vi "Handle Command.vi"(8 "error in (no error)":errorcluster, 9 "params in":variant, 10 "command":string, 11 "Instrument in":refnum<class "Instrument.lvclass">) -> (0 "error out":errorcluster, 1 "processed data":variant, 2 "command out":string, 3 "Instrument out":refnum<class "Instrument.lvclass">)   [LabVIEW 2019, in "Instrument.lvlib" / "Instrument.lvclass"]
doc: "Override to add additional commands supported by your Instrument."
uses:
  Instrument.lvclass
  Typedefs/Instrument.Commands--Enum.ctl
  Typedefs/Instrument.ProtectedCommands--Enum.ctl
  Typedefs/Instrument.SET--cluster.ctl
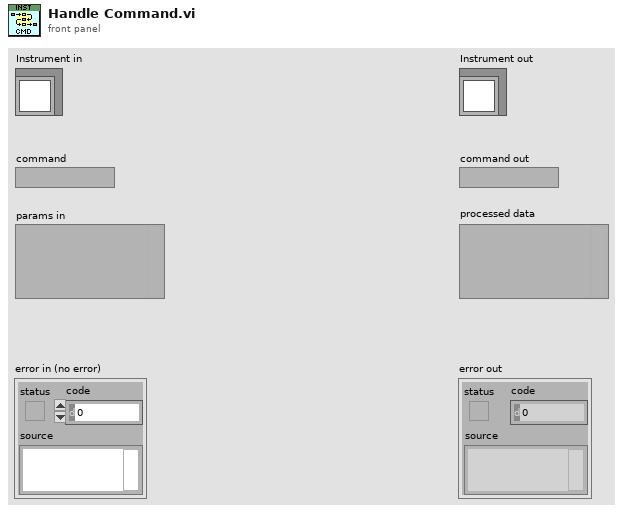
[diagram p1: front panel]
types:
  T1 = typedef "Instrument.lvlib/Instrument.lvclass/Instrument.ProtectedCommands--Enum.ctl" = enum16{"setConfiguration", "setIDN", "setAll", "setAllData"}
  T2 = typedef "Instrument.lvlib/Instrument.lvclass/Instrument.Commands--Enum.ctl" = enum16{"ACK", "HELP", "IDN", "getAll", "getAllData"}
  T3 = typedef "Instrument.lvlib/Instrument.lvclass/Instrument.SET--cluster.ctl" = cluster{"parameter":string, "Data":variant}
  T4 = typedef "Instrument.lvlib/Instrument.lvclass/Instrument.IDN--cluster.ctl" = cluster{"vendor":string, "model":string, "serial":string, "firmware":string}
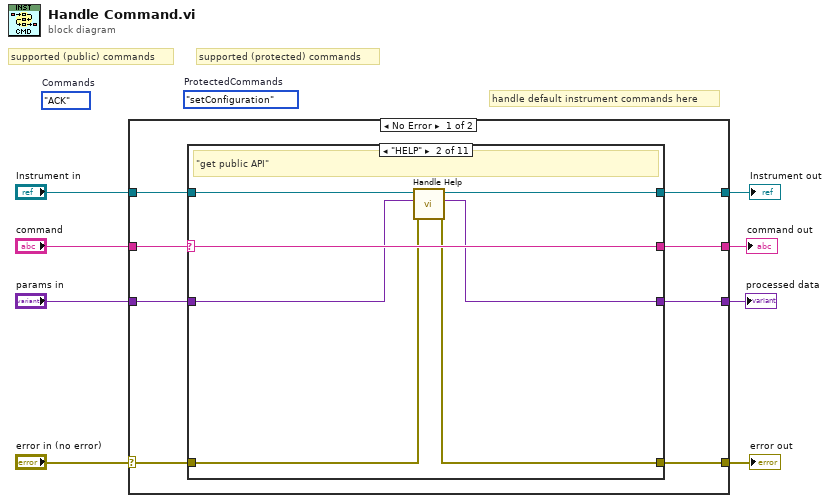
[diagram p0: block diagram]
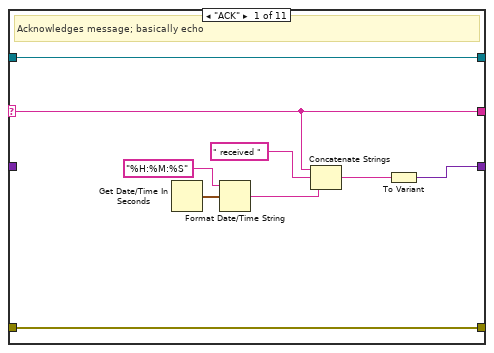
[diagram p2: hidden frame]
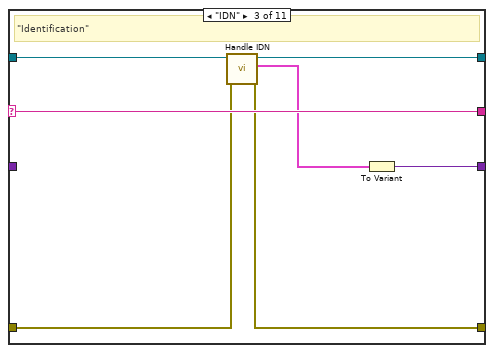
[diagram p3: hidden frame]
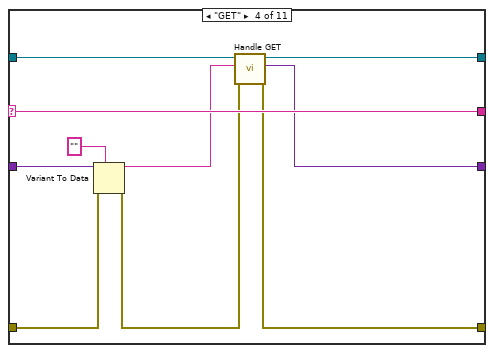
[diagram p4: hidden frame]
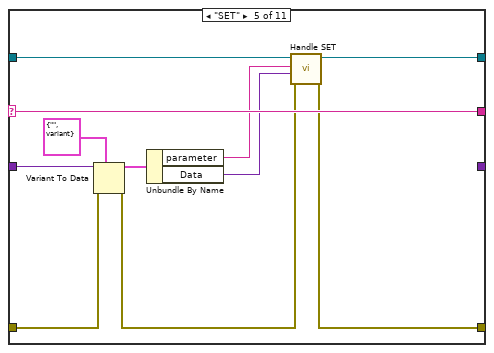
[diagram p5: hidden frame]
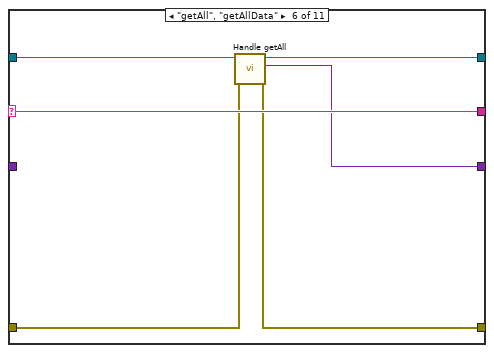
[diagram p6: hidden frame]
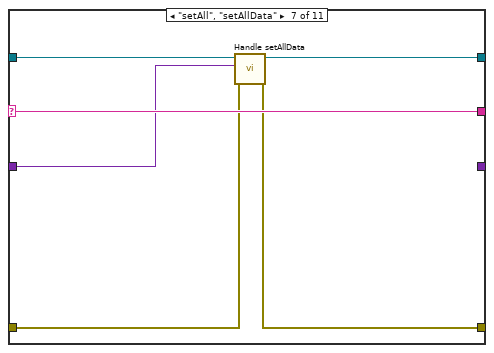
[diagram p7: hidden frame]
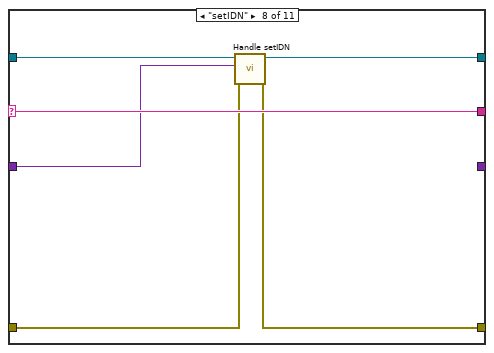
[diagram p8: hidden frame]
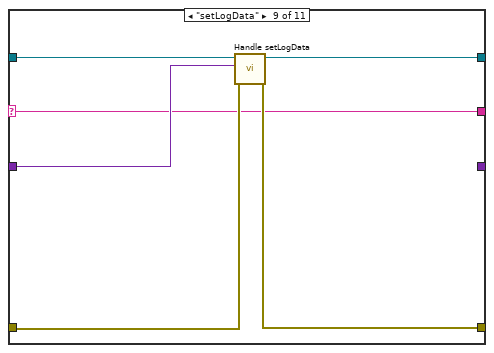
[diagram p9: hidden frame]
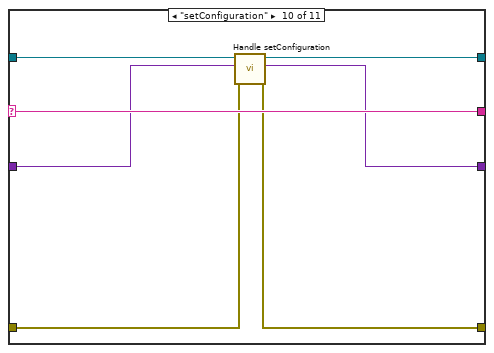
[diagram p10: hidden frame]
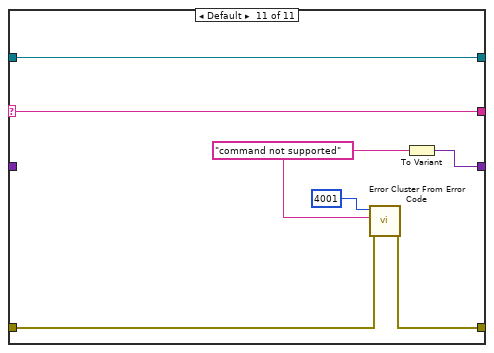
[diagram p11: hidden frame]
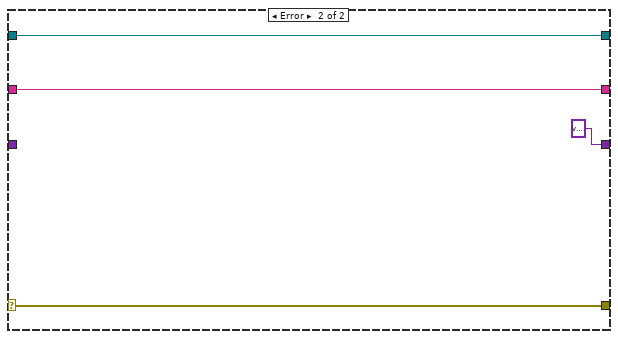
[diagram p12: hidden frame]
diagram:
  (unwired) Instrument.ProtectedCommands--Enum."setConfiguration"  # ProtectedCommands
  (unwired) Instrument.Commands--Enum."ACK"  # Commands
  # "supported (protected) commands"
  # "supported (public) commands"
  # "handle default instrument commands here"
  n1 = case shown="No Error" "error in (no error)" {
    selector: "error in (no error)" -> [w13 w101]
    tunnel: [w12 w101] -> w7
    tunnel: [w15 w100] -> w5
    tunnel: "Instrument in" -> [w16 w100]
    tunnel: "command" -> [w10 w99]
    tunnel: [w14 variant ("error message (\"\")")] -> w4
    tunnel: "params in" -> [w9 _]
    tunnel: [w11 w99] -> w1
    frame No Error {
      n2 = case shown="\"HELP\"" w10 {
        selector: w10 -> [w19 w30 w39 w49 w60 w66 w72 w78 w79 w90 w95]
        tunnel: w16 -> [w25 w32 w36 w47 w58 w63 w71 w76 w84 w87 w97]
        tunnel: [w25 w31 w37 w48 w59 w62 w70 w74 w83 w86 w97] -> w15
        tunnel: [w17 w27 w38 w45 _ w61 _ _ _ w85 w96] -> w14
        tunnel: w13 -> [w22 w29 w33 w41 w53 w65 w69 w77 w81 w89 w93]
        tunnel: [w22 w28 w34 w46 w57 w64 w68 w75 w80 w88 w92] -> w12
        tunnel: [w19 w30 w39 w49 w60 w66 w72 w78 w79 w90 w95] -> w11
        tunnel: w9 -> [_ w26 _ w43 w55 _ w67 w73 w82 w85 _]
        frame "ACK" {
          # "Acknowledges message; basically echo"
          n3 = Get Date/Time In Seconds() -> (seconds since 1Jan1904=w23:timestamp)
          n4 = Format Date/Time String(time format string (%c)="%H:%M:%S", seconds (now)=w23) -> (date/time string=w24:string)  [unwired: 1 in]
          n5 = Concatenate Strings(w19, " received " ("data"), w24) -> (w21:string)
          n6 = To Variant(anything=w21) -> (Variant=w17:variant)
        }
        frame "HELP" {
          # "\"get public API\""
          n7 = call "Handle Help.vi"("error in (no error)"=w29, "Command"=w26, "Instrument in"=w32) -> ("error out"=w28:errorcluster, "Help"=w27:variant, "Instrument out"=w31:refnum<class "Instrument.lvclass">)  [unwired: 6 in]
        }
        frame "IDN" {
          # "\"Identification\""
          n8 = call "Handle IDN.vi"("error in (no error)"=w33, "Instrument in"=w36) -> ("error out"=w34:errorcluster, "IDN"=w35:T4, "Instrument out"=w37:refnum<class "Instrument.lvclass">)  [unwired: 7 in]
          n9 = To Variant(anything=w35) -> (Variant=w38:variant)
        }
        frame "GET" {
          n10 = Variant To Data(error in=w41, type="", Variant=w43) -> (data=w40:string, error out=w42:errorcluster)
          n11 = call-dynamic "Handle GET.vi"("error in (no error)"=w42, "parameter"=w40, "Instrument in"=w47) -> ("error out"=w46:errorcluster, "data out"=w45:variant, "Instrument out"=w48:refnum<class "Instrument.lvclass">)  [unwired: 6 in]
        }
        frame "SET" {
          n12 = Variant To Data(error in=w53, type=T3 {"parameter"="", "Data"=variant} ("GETSET"), Variant=w55) -> (data=w52:T3, error out=w54:errorcluster)
          n13 = Unbundle By Name(w52) -> ("parameter"=w51:string, "Data"=w50:variant)
          n14 = call-dynamic "Handle SET.vi"("error in (no error)"=w54, "data"=w50, "parameter"=w51, "Instrument in"=w58) -> ("error out"=w57:errorcluster, "Instrument out"=w59:refnum<class "Instrument.lvclass">)  [unwired: 5 in, 1 out]
        }
        frame "getAll", "getAllData" {
          n15 = call-dynamic "Handle getAll.vi"("error in (no error)"=w65, "Instrument in"=w63) -> ("error out"=w64:errorcluster, "getAll"=w61:variant, "Instrument out"=w62:refnum<class "Instrument.lvclass">)  [unwired: 7 in]
        }
        frame "setAll", "setAllData" {
          n16 = call-dynamic "Handle setAllData.vi"("error in (no error)"=w69, "AllData"=w67, "Instrument in"=w71) -> ("error out"=w68:errorcluster, "Instrument out"=w70:refnum<class "Instrument.lvclass">)  [unwired: 7 in]
        }
        frame "setIDN" {
          n17 = call "Handle setIDN.vi"("error in (no error)"=w77, "IDN"=w73, "Instrument in"=w76) -> ("error out"=w75:errorcluster, "Instrument out"=w74:refnum<class "Instrument.lvclass">)  [unwired: 7 in]
        }
        frame "setLogData" {
          n18 = call "Handle setLogData.vi"("error in (no error)"=w81, "LogData"=w82, "Instrument in"=w84) -> ("error out"=w80:errorcluster, "Instrument out"=w83:refnum<class "Instrument.lvclass">)  [unwired: 7 in]
        }
        frame "setConfiguration" {
          n19 = call-dynamic "Handle setConfiguration.vi"("error in (no error)"=w89, "setConfiguration"=w85, "Instrument in"=w87) -> ("error out"=w88:errorcluster, "Instrument out"=w86:refnum<class "Instrument.lvclass">)  [unwired: 7 in]
        }
        frame Default {
          w91 = "command not supported" ("error message (\"\")")
          n20 = call <vilib>:"Error Cluster From Error Code.vi"("error in (no error)"=w93, "error message (\"\")"=w91, "error code (0)"=4001) -> ("error out"=w92:errorcluster)  [unwired: 6 in]
          n21 = To Variant(anything=w91) -> (Variant=w96:variant)
        }
      }
    }
    frame Error {
    }
  }
  "error out" <- w7
  "Instrument out" <- w5
  "processed data" <- w4
  "command out" <- w1
